vi "GetVIsWithCompiledCode.vi"(8 "error in (no error)":errorcluster, 11 "Search Path":path) -> (0 "error out":errorcluster, 3 "VIs with compiled code":path[](array[path]))   [LabVIEW 2015, in "VeriStandTestUtilities.lvlib"]
uses:
  VeriStandTestUtilities.lvlib
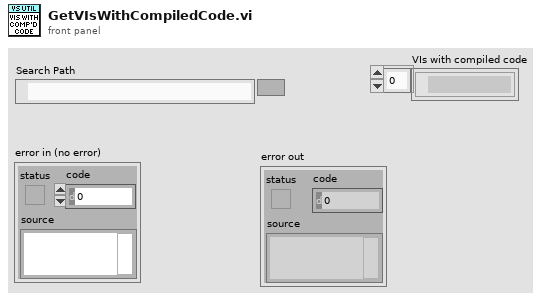
[diagram p1: front panel]
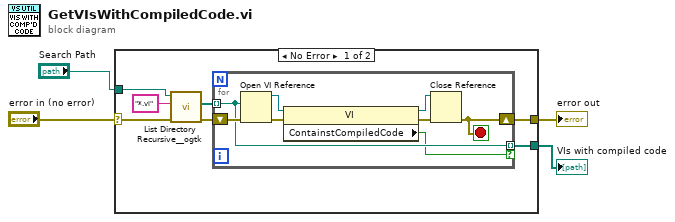
[diagram p0: block diagram]
diagram:
  n1 = case shown="No Error" "error in (no error)" {
    selector: "error in (no error)" -> [w6 w20]
    tunnel: [w8 w20] -> w4
    tunnel: "Search Path" -> [w10 _]
    tunnel: [w5 _] -> w1
    frame No Error {
      n2 = call <userlib>:"List Directory Recursive__ogtk.vi"("error in (no error)"=w6, "pattern"="*.vi", "Path"=w10) -> ("error out"=w7:errorcluster, "file paths"=w9:path[])  [unwired: 5 in, 2 out]
      n3 = for {
        tunnel: w9 -> [w14] mode=indexing
        shift-right: [w12] -> w8
        shift-left: w7 -> [w19]
        tunnel: [w14] -> w5 mode=indexing if=w13
        stop <- w12 stop-if-true
        n4 = Open VI Reference(vi path=w14, error in (no error)=w19) -> (vi reference=w15:refnum<vi>, error out=w18:errorcluster)  [unwired: 4 in]
        n5 = property class="VI"(reference=w15, error in=w18) -> (reference out=w16:refnum<vi>, error out=w17:errorcluster, "ContainstCompiledCode"=w13:bool)
        n6 = Close Reference(reference=w16, error in (no error)=w17) -> (error out=w12:errorcluster)
      }
    }
    frame Error {
    }
  }
  "error out" <- w4
  "VIs with compiled code" <- w1
